vi "LV_OPC_Test_Net.vi"() -> ()   [LabVIEW 2024]
uses:
  C:/Users/Andrey/Desktop/LV_OPC-Client-x64/LV_OPC_Test/OPC.NET/OpcNetApi.dll
  OPC.NET/OpcNetApi.dll
  OPC.NET/LV_OPC_NET.lvlib
panel:
  out "Value DBL":dbl=3.0
  out "Value SGL":sgl=0.1
  out "server status":T1={"CurrentTime"=timestamp(3795340254.486 s since 1904-01-01), "LastUpdateTime"=timestamp(0 s since 1904-01-01), "ProductVersion"="3.0.0", "ServerState"=1, "StartTime"=timestamp(3795340254.446 s since 1904-01-01), "StatusInfo"="The server is running normally.", "VendorInfo"="Tagger's OPC"}
  out "server properties":T2={"Filters"=9, "IsConnected"=TRUE, "Locale"="", "Name"="National Instruments.Variable Engine.1", "Subscriptions"=refnum, "SupportedLocales"=["en-US"], "Url"=refnum}
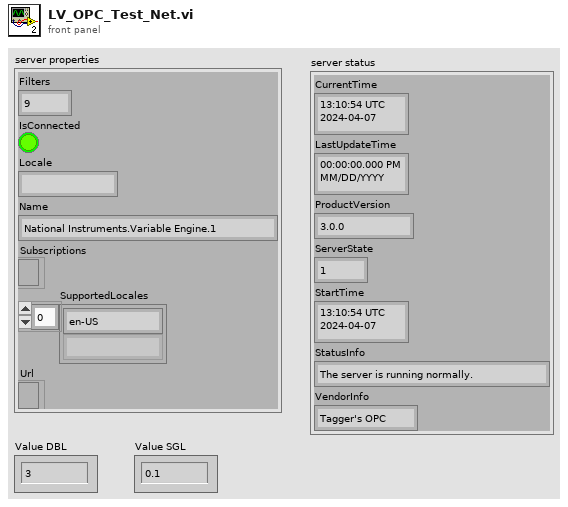
[diagram p1: front panel]
types:
  T1 = cluster{"CurrentTime":timestamp, "LastUpdateTime":timestamp, "ProductVersion":string, "ServerState":i32, "StartTime":timestamp, "StatusInfo":string, "VendorInfo":string}
  T2 = cluster{"Filters":i32, "IsConnected":bool, "Locale":string, "Name":string, "Subscriptions":refnum<k24>, "SupportedLocales":string[], "Url":refnum<k24>}
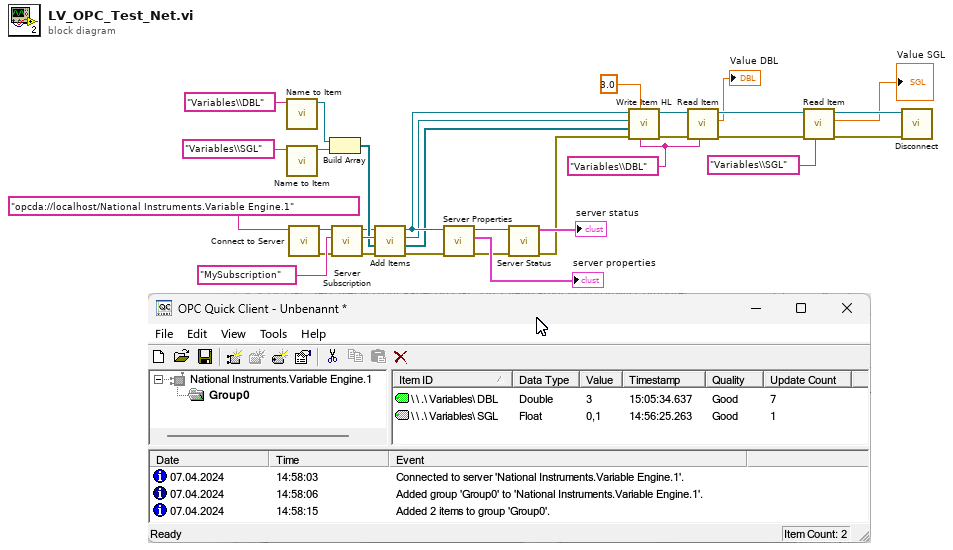
[diagram p0: block diagram]
diagram:
  w13 = "Variables\\DBL" ("itemName")
  n1 = call "Name to Item.vi"("itemName"="Variables\\DBL") -> (".NET Refnum out"=w27:refnum<k24>)  [unwired: 9 in, 1 out]
  n2 = call "Name to Item.vi"("itemName"="Variables\\SGL") -> (".NET Refnum out"=w11:refnum<k24>)  [unwired: 9 in, 1 out]
  n3 = call "Connect to Server.vi"("url"="opcda://localhost/National Instruments.Variable Engine.1") -> ("error out"=w18:errorcluster, ".NET Refnum out"=w29:refnum<k24>)  [unwired: 9 in]
  n4 = Build Array(w27, w11) -> (w26:refnum<k24>[])
  n5 = call "Server Subscription.vi"("error in (no error)"=w18, "Name"="MySubscription", ".NET Refnum in"=w29) -> ("error out"=w19:errorcluster, "CreateSubscription"=w28:refnum<k24>, ".NET Refnum out"=w15:refnum<k24>)  [unwired: 6 in]
  n6 = call "Add Items.vi"("error in (no error)"=w19, "Array"=w26, "CreateSubscription in"=w28, ".NET Refnum in"=w15) -> ("error out"=w21:errorcluster, "AddItems"=w7:refnum<k24>[], "CreateSubscription out"=w8:refnum<k24>, ".NET Refnum out"=w9:refnum<k24>)  [unwired: 4 in]
  n7 = call "Server Properties.vi"("error in (no error)"=w21, ".NET Refnum in"=w9) -> ("error out"=w20:errorcluster, "Cluster"=→"server properties":T2, ".NET Refnum out"=w24:refnum<k24>)  [unwired: 7 in]
  n8 = call "Server Status.vi"("error in (no error)"=w20, ".NET Refnum in"=w24) -> ("error out"=w12:errorcluster, "Cluster"=→"server status":T1)  [unwired: 8 in]
  n9 = call "Write Item HL.vi"("itemName"=w13, "Numeric"=sgl 3.0, "error in"=w12, "AddItems"=w7, "CreateSubscription in"=w8, ".Server Refnum in"=w9) -> ("error out"=w14:errorcluster, ".NET Refnum out"=w32:refnum<k24>)  [unwired: 3 in, 1 out]
  n10 = call "Read Item.vi"("itemName"=w13, "error in (no error)"=w14, ".NET Refnum in"=w32) -> ("error out"=w4:errorcluster, "Value (SGL/DBL only!)"=→"Value DBL":dbl, ".NET Refnum out"=w6:refnum<k24>)  [unwired: 2 in, 4 out]
  n11 = call "Read Item.vi"("itemName"="Variables\\SGL", "error in (no error)"=w4, ".NET Refnum in"=w6) -> ("error out"=w3:errorcluster, "Value (SGL/DBL only!)"=→"Value SGL":dbl, ".NET Refnum out"=w5:refnum<k24>)  [unwired: 2 in, 4 out]
  n12 = call "Disconnect.vi"("error in (no error)"=w3, ".NET Refnum in"=w5) -> ()  [unwired: 10 in]
